vi "MCCShutter.vi"(0 "MCCPMT in":refnum<class "MCCPMT.lvclass">, 11 "error in (no error)":errorcluster) -> (4 "MCCPMT out":refnum<class "MCCPMT.lvclass">, 15 "error out":errorcluster)   [LabVIEW 2012, in "MCCPMT.lvclass"]
uses:
  MCCPMT.lvclass
  <vilib>/ULx/Create Channel.llb/ULx Create Channel (DO-Digital Output).vi
  <vilib>/ULx/Write.llb/ULx Write (Digital Bool 1Line 1Point).vi
panel:
  in  "lines":refnum<k21>
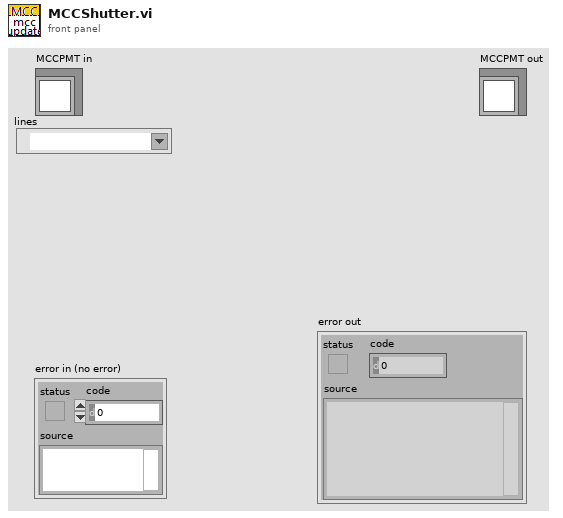
[diagram p1: front panel]
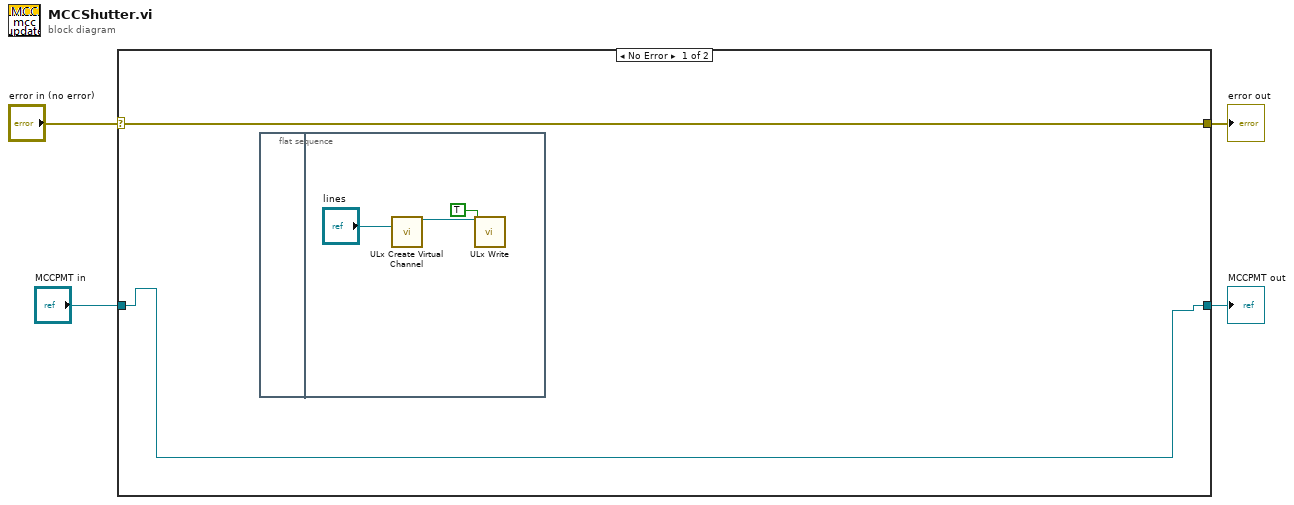
[diagram p0: block diagram]
diagram:
  n1 = case shown="No Error" "error in (no error)" {
    selector: "error in (no error)" -> [w6 w11]
    tunnel: [w6 w11] -> w3
    tunnel: [w5 w10] -> w1
    tunnel: "MCCPMT in" -> [w5 w10]
    frame No Error {
      n2 = flat-sequence {
        frame #0 {
        }
        frame #1 {
          n3 = call-poly <vilib>:"ULx Create Virtual Channel.vi"("lines"="lines") -> ("task out"=w9:refnum<k24>)  [unwired: 13 in, 1 out]
          n4 = call-poly <vilib>:"ULx Write.vi"("task in"=w9, "data"=TRUE) -> ()  [unwired: 11 in, 3 out]
        }
      }
    }
    frame Error {
    }
  }
  "error out" <- w3
  "MCCPMT out" <- w1
